vi "Get Serial Number.vi"(8 "error in (no error)":errorcluster, 11 "Device ID (0)":i32) -> (0 "error out":errorcluster, 1 "Head Serial No.":string, 2 "Controller Serial No.":string, 3 "Device ID out":i32)   [LabVIEW 2015, in "KEYENCE LJ-X8000A.lvlib"]
doc: "This function gets the serial numbers."
uses:
  KEYENCE LJ-X8000A.lvlib
panel:
  # "(c) 2019 KEYENCE CORPORATION.  ALL RIGHTS RESERVED."
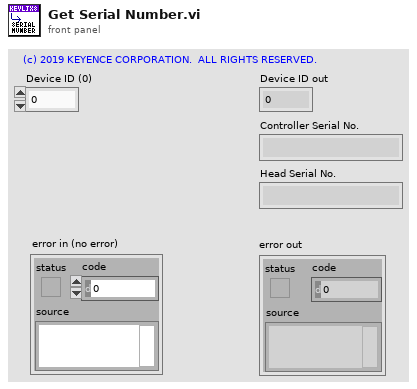
[diagram p1: front panel]
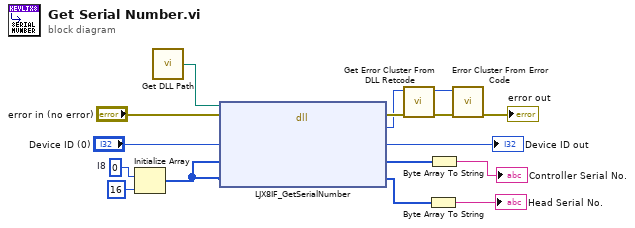
[diagram p0: block diagram]
diagram:
  w9 = i8 0  # I8
  n1 = Initialize Array(w9, 16 ("次元サイズ")) -> (w7:i8[])
  n2 = call "Get DLL Path.vi"() -> ("DLL Path"=w13:path)  [unwired: 3 in]
  n3 = dll-call lib="C:/Program Files (x86)/National Instruments/LabVIEW 2018/instr.lib/KEYENCE LJ-X8000/LJX8_IF.*" fn="LJX8IF_GetSerialNumber"(path in=w13, error in="error in (no error)", "lDeviceId"="Device ID (0)", "pControllerSerialNo"=w7, "pHeadSerialNo"=w7) -> (error out=w11:errorcluster, "lRetCode"=w10:i32, "lDeviceId"=→"Device ID out":i32, "pControllerSerialNo"=w6:i8[], "pHeadSerialNo"=w5:i8[])  [unwired: 1 in, 1 out]
  n4 = call "Get Error Cluster From DLL Retcode.vi"("error in (no error)"=w11, "DLL Return Code"=w10) -> ("error out"=w12:errorcluster, "VI Error Code"=w1:i32)  [unwired: 8 in]
  n5 = Byte Array To String(unsigned byte array=w5) -> (string=→"Head Serial No.":string)
  n6 = Byte Array To String(unsigned byte array=w6) -> (string=→"Controller Serial No.":string)
  n7 = call <vilib>:"Error Cluster From Error Code.vi"("error in (no error)"=w12, "error code (0)"=w1) -> ("error out"=→"error out":errorcluster)  [unwired: 7 in]
